vi "OPC Write.vi"(8 "error in (no error)":errorcluster, 10 "Mode":T1=enum."Initialize", 11 "OPC Server":string="opc://localhost/RSLinx OPC Server/[ML1400]") -> (0 "error out":errorcluster, 2 "data ref":refnum<k13>[](array[refnum]), 3 "all ref":refnum<k13>[](array[refnum]))   [LabVIEW 2019]
doc: "This VI reads multiple OPC items at one time. Specify which items you want to read or use the predetermined list of items. The predetermined list of items specifies items from the National Instruments.OPCDemo server, which has been installed on your machine."
uses:
  Write Mode.ctl
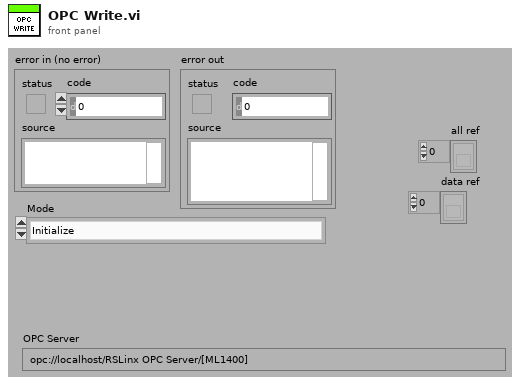
[diagram p1: front panel]
types:
  T1 = typedef "Write Mode.ctl" = enum16{"GetRef", "Initialize", "Close"}
  T2 = enum16{"Read", "Write", "ReadWrite", "BufferedRead", "BufferedReadWrite"}
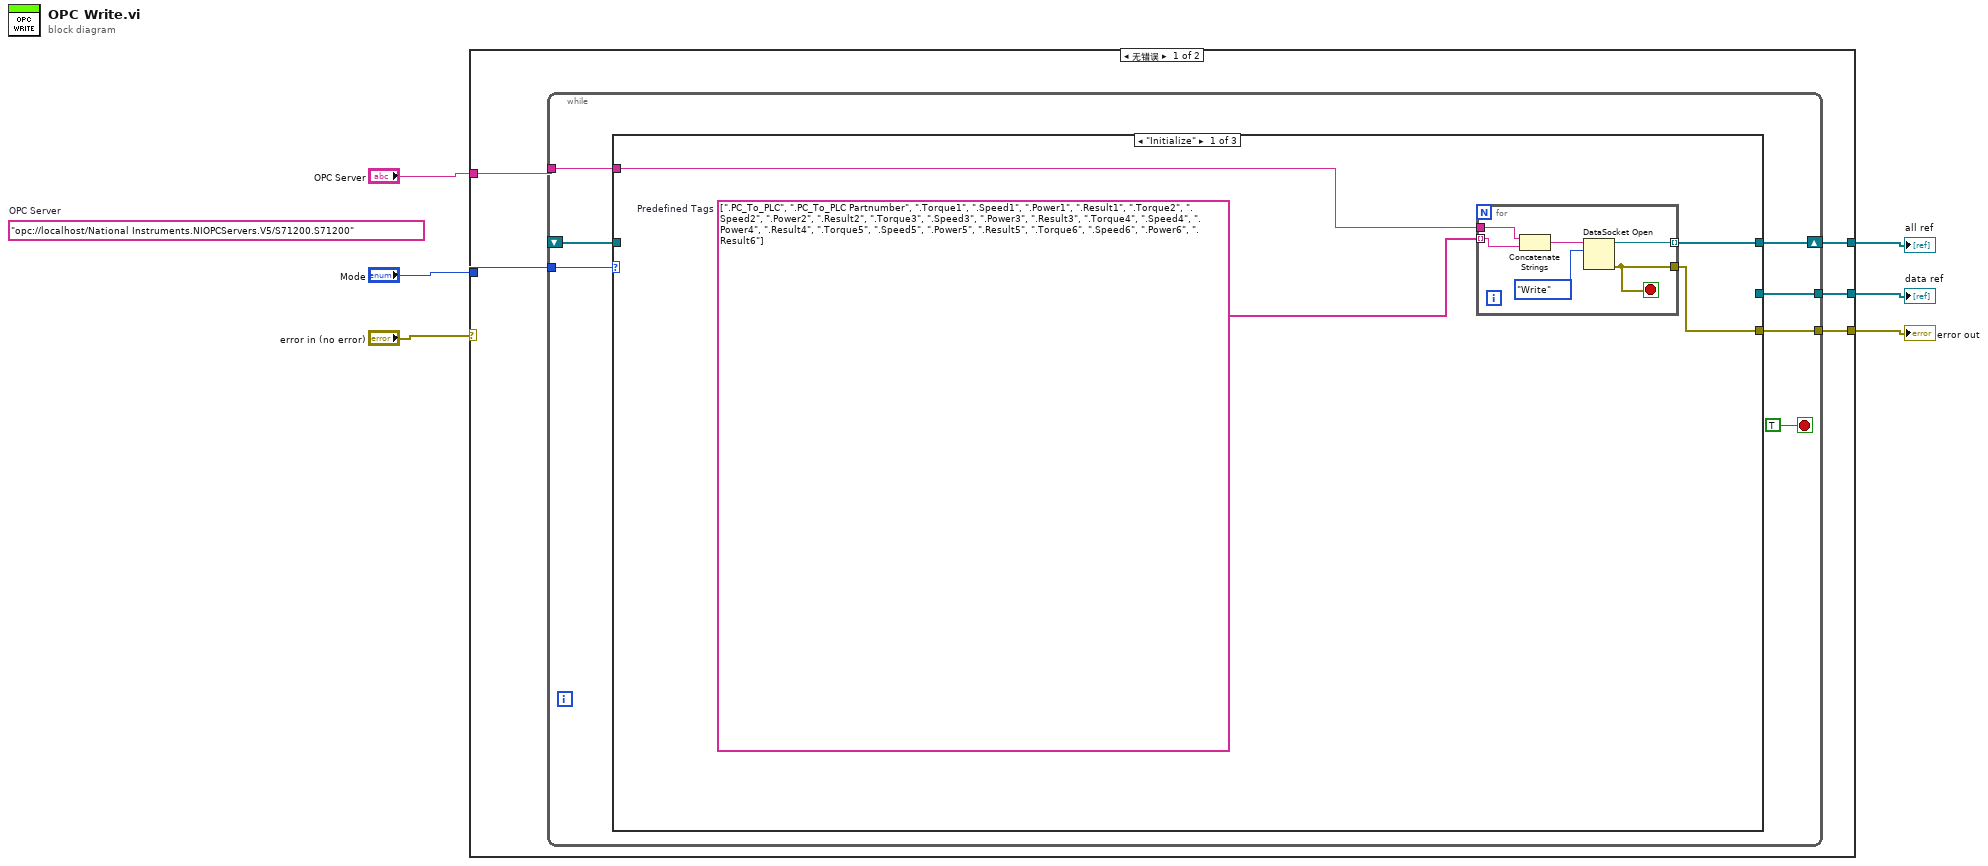
[diagram p0: block diagram]
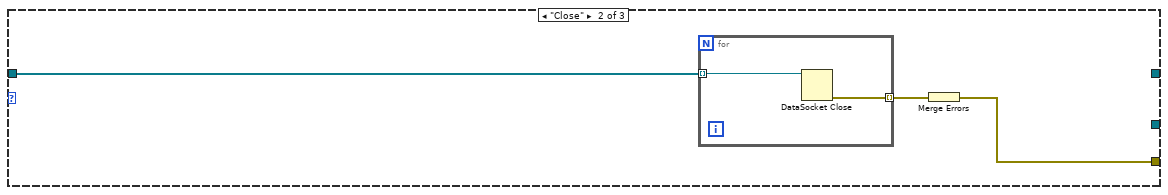
[diagram p2: hidden frame]
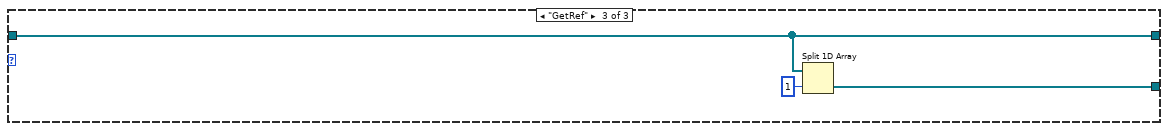
[diagram p3: hidden frame]
diagram:
  (unwired) "opc://localhost/National Instruments.NIOPCServers.V5/S71200.S71200"  # OPC Server
  n1 = case shown="无错误" "error in (no error)" {
    selector: "error in (no error)" -> [_ w37]
    tunnel: "Mode" -> [w11 _]
    tunnel: [w10 w37] -> w5
    tunnel: "OPC Server" -> [w9 _]
    tunnel: [w8 _] -> w4
    tunnel: [w7 _] -> w3
    frame No Error {
      n2 = while {
        shift-right: [w17] -> w8
        shift-left: _ -> [w14]
        tunnel: [w15] -> w10
        tunnel: w9 -> [w13]
        tunnel: [w12] -> w7
        tunnel: w11 -> [w16]
        stop <- TRUE stop-if-true
        n3 = case shown="\"Initialize\"" w16 {
          tunnel: [w22 _ w34] -> w17
          tunnel: [w21 w29 _] -> w15
          tunnel: w14 -> [_ w31 w34]
          tunnel: w13 -> [w20 _ _]
          tunnel: [_ _ w35] -> w12
          frame "Initialize" {
            w19 = string[] [".PC_To_PLC", ".PC_To_PLC Partnumber", ".Torque1", ".Speed1", ".Power1", ".Result1", ".Torque2", ".Speed2", ".Power2", ".Result2", ".Torque3", ".Speed3", ".Power3", ".Result3", ".Torque4", ".Speed4", ".Power4", ".Result4", ".Torque5", ".Speed5", ".Power5", ".Result5", ".Torque6", ".Speed6", ".Power6", ".Result6"]  # Predefined Tags
            n4 = for {
              tunnel: w19 -> [w24] mode=indexing
              tunnel: w20 -> [w25]
              tunnel: [w26] -> w22 mode=indexing
              tunnel: [w23] -> w21
              stop <- w23 stop-if-true
              n5 = Concatenate Strings(w25, w24) -> (w27:string)
              n6 = DataSocket Open(10:T2."Write" ("mode"), 11:w27) -> (0:w23:errorcluster, 3:w26:refnum<k13>)  [unwired: 1 in, 1 out]
            }
          }
          frame "Close" {
            n7 = for {
              tunnel: [w33] -> w30 mode=indexing
              tunnel: w31 -> [w32] mode=indexing
              n8 = DataSocket Close(11:w32) -> (0:w33:errorcluster)  [unwired: 2 in, 1 out]
            }
            n9 = Merge Errors(w30) -> (w29:errorcluster)
          }
          frame "GetRef" {
            n10 = Split 1D Array(array=w34, index=1) -> (second subarray=w35:refnum<k13>[])  [unwired: 1 out]
          }
        }
      }
    }
    frame Error {
    }
  }
  "error out" <- w5
  "all ref" <- w4
  "data ref" <- w3
